vi "Convert_to_2009.vi"(8 "error in (no error)":errorcluster, 11 "IB_RegDest in":refnum<class "IB_RegDest.lvclass">) -> (0 "error out":errorcluster, 2 "preserve?":bool, 3 "RegDest":T1)   [LabVIEW 2020, in "IB_RegDest.lvclass"]
uses:
  <vilib>/AppBuilder/IB_Classes/RegDest/IB_RegDest.lvclass
  <vilib>/AppBuilder/IB_Classes/RegDest/IB_RegDest.lvclass/IB_RegDest.ctl
  <resource>/Framework/Providers/Builds/Installer/CDK_sTypeDef_DirInfo.ctl
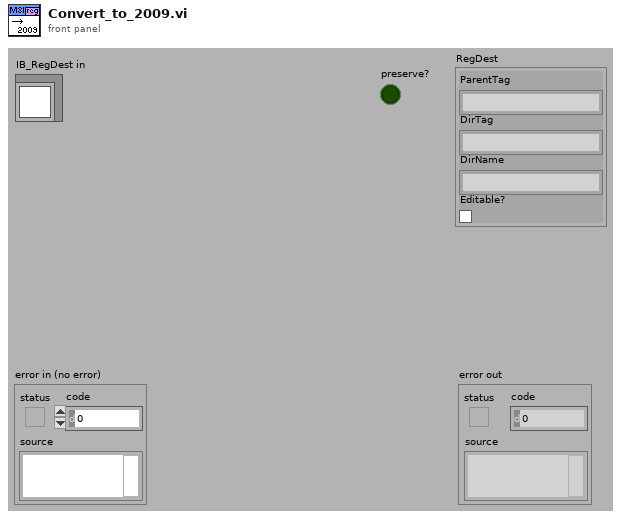
[diagram p1: front panel]
types:
  T1 = typedef "CDK_sTypeDef_DirInfo.ctl" = cluster{"ParentTag":string, "DirTag":string, "DirName":string, "Editable?":bool}
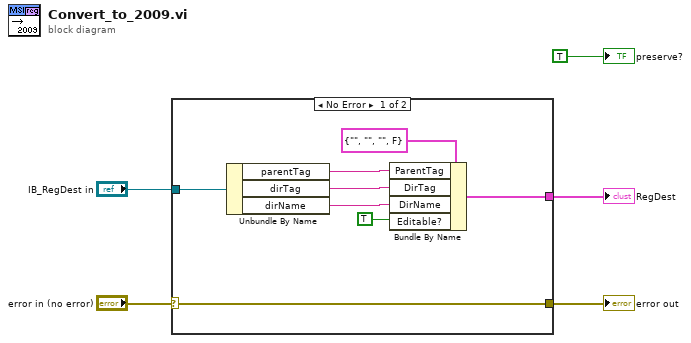
[diagram p0: block diagram]
diagram:
  n1 = case shown="No Error" "error in (no error)" {
    selector: "error in (no error)" -> [w13 w14]
    tunnel: [w13 w14] -> w4
    tunnel: "IB_RegDest in" -> [w7 _]
    tunnel: [w6 _] -> w2
    frame No Error {
      n2 = Unbundle By Name(w7) -> ("parentTag"=w12:string, "dirTag"=w10:string, "dirName"=w11:string)
      n3 = Bundle By Name(cluster=T1 {"ParentTag"="", "DirTag"="", "DirName"="", "Editable?"=FALSE} ("DirInfo"), "ParentTag"=w12, "DirTag"=w10, "DirName"=w11, "Editable?"=TRUE) -> (w6:T1)
    }
    frame Error {
    }
  }
  "error out" <- w4
  "RegDest" <- w2
  "preserve?" <- TRUE
